vi "AddPropertyUnscale.vi"(0 "Data":T1={"Ref Cluster"={"String"=refnum, "U8"=refnum, "I8"=refnum, "U32"=refnum, "I32"=refnum, "U64"=refnum, "I64"=refnum, "Ring"=refnum, "DBL"=refnum, "Add"=refnum, "Remove"=refnum, "Property tree"=refnum}, "JSON Text"="", "Original JSON Text"="", "Caps"={"properties"=[], "physical channels"=[], "registers"=[], "scales"=[], "enums"=[], "productName"=""}, "SLSC Output Tree"=[], "Ref Index and Control Type"={"index"=0, "Datatype"=""}, "Selected Type and name"={"Selected Type"=enum."Property", "Selected Property Name"="Device/Properties/NI.Debug.ScratchU32.Min10Max20"}, "Update whole Tree?"=FALSE}, 1 "Scale method":string, 2 "Bitfield":string="DebugScratch8/ScratchI8", 5 "error in":errorcluster, 6 "Type&Value":cluster{"type":string, "Variant":variant}) -> (14 "Variant":variant, 19 "error out":errorcluster)   [LabVIEW 2017]
uses:
  <vilib>/Utility/Data Type/NI_Data Type.lvlib
  Ctrl/TableScale.ctl
  API/Scale/Scale.lvlib
  Ctrl/Coercion.ctl
  Ctrl/PolynomialScale.ctl
  Ctrl/LinearScale.ctl
  API/Bitfield/Bitfield.lvlib
  API/Scale/Unscale(Linear).vi
  API/Scale/Unscale(Table).vi
  API/Scale/Unscale(Polynomial).vi
  Ctrl/ScaleType.ctl
  Ctrl/Property.ctl
  Ctrl/PhysicalChannel.ctl
  Ctrl/Bitfield.ctl
  Ctrl/Register.ctl
  Ctrl/Scale.ctl
  Ctrl/EnumValue.ctl
  Ctrl/Enum.ctl
  Ctrl/Caps.ctl
  Ctrl/Data.ctl
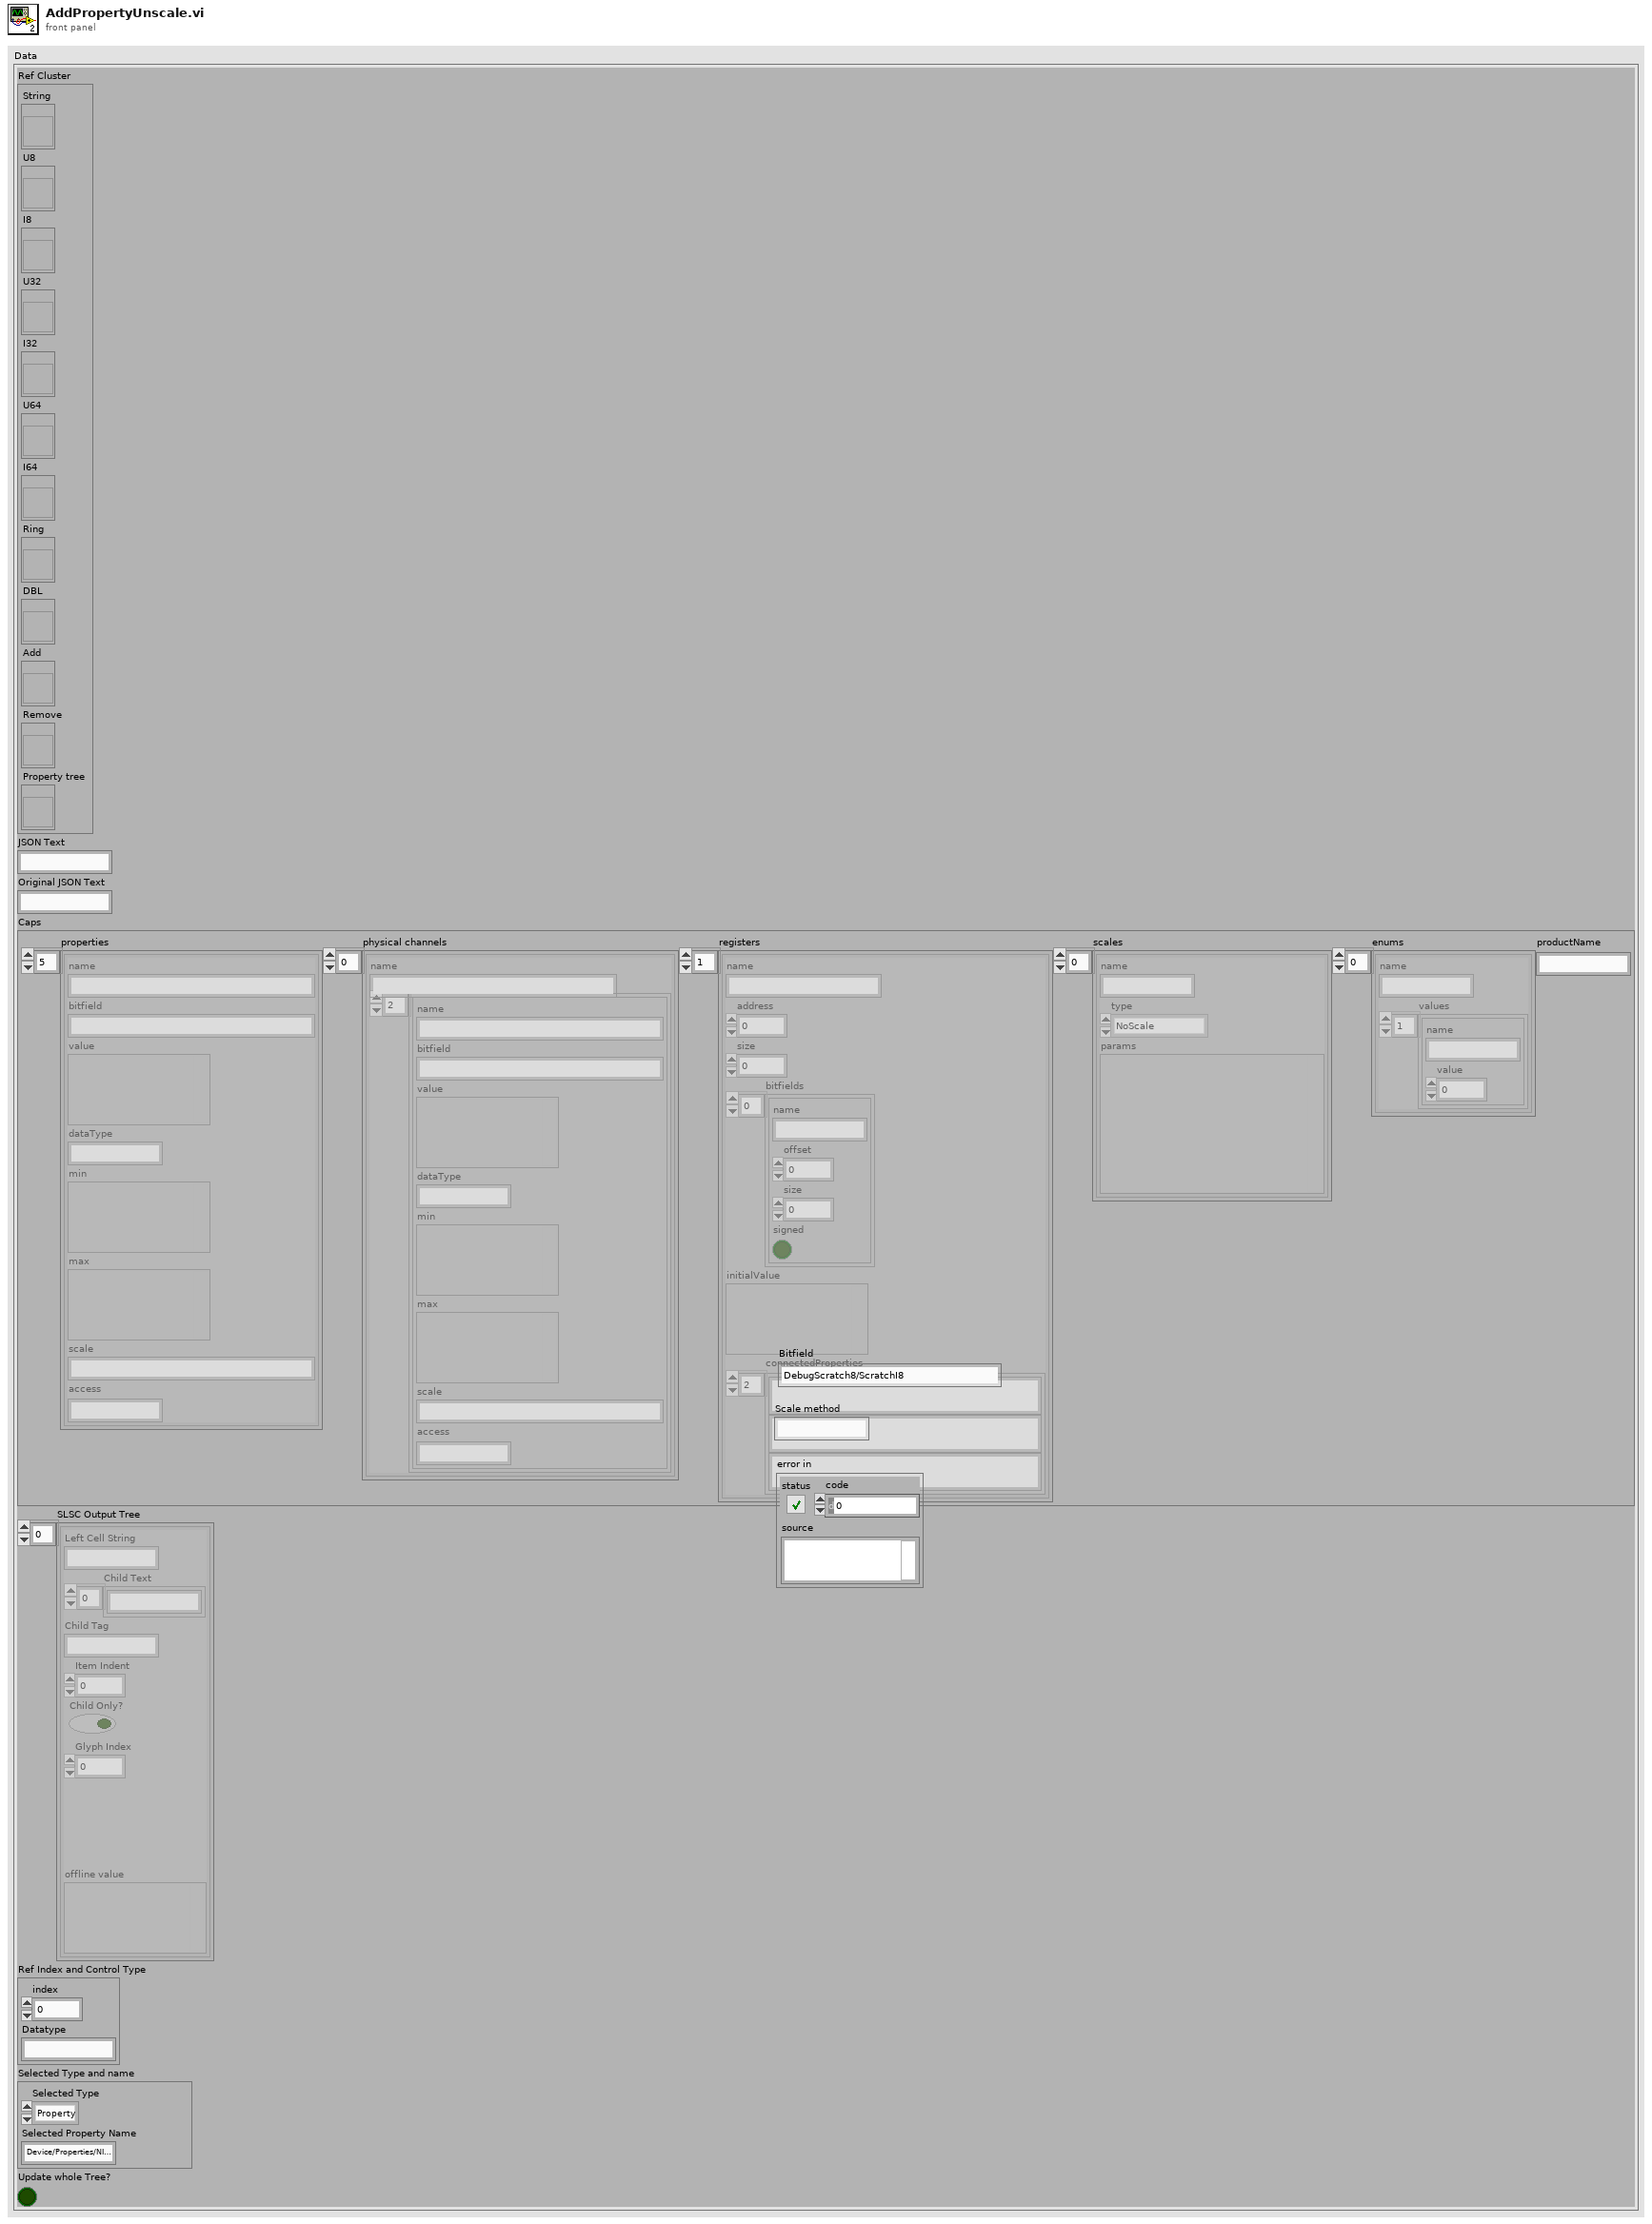
[diagram p1: front panel]
types:
  T1 = typedef "Data.ctl" = cluster{"Ref Cluster":cluster{"String":refnum<vi>, "U8":refnum<vi>, "I8":refnum<vi>, "U32":refnum<vi>, "I32":refnum<vi>, "U64":refnum<vi>, "I64":refnum<vi>, "Ring":refnum<vi>, "DBL":refnum<vi>, "Add":refnum<vi>, "Remove":refnum<vi>, "Property tree":refnum<vi>}, "JSON Text":string, "Original JSON Text":string, "Caps":T2, "SLSC Output Tree":cluster{"Left Cell String":string, "Child Text":string[], "Child Tag":string, "Item Indent":i32, "Child Only?":bool, "Glyph Index":i32, "offline value":variant}[], "Ref Index and Control Type":cluster{"index":i32, "Datatype":string}, "Selected Type and name":cluster{"Selected Type":enum16{"Property", "Physical Channel", "Other"}, "Selected Property Name":string}, "Update whole Tree?":bool}
  T2 = typedef "Caps.ctl" = cluster{"properties":T3[], "physical channels":T4[], "registers":T5[], "scales":T7[], "enums":T9[], "productName":string}
  T3 = typedef "Property.ctl" = cluster{"name":string, "bitfield":string, "value":variant, "dataType":string, "min":variant, "max":variant, "scale":string, "access":string}
  T4 = typedef "PhysicalChannel.ctl" = cluster{"name":string, "properties":T3[]}
  T5 = typedef "Register.ctl" = cluster{"name":string, "address":i32, "size":i32, "bitfields":T6[], "initialValue":variant, "connectedProperties":string[]}
  T6 = typedef "Bitfield.ctl" = cluster{"name":string, "offset":i32, "size":i32, "signed":bool}
  T7 = typedef "Scale.ctl" = cluster{"name":string, "type":T8, "params":variant}
  T8 = typedef "ScaleType.ctl" = enum16{"NoScale", "Table", "Polynomial", "Linear"}
  T9 = typedef "Enum.ctl" = cluster{"name":string, "values":T10[]}
  T10 = typedef "EnumValue.ctl" = cluster{"name":string, "value":i32}
  T11 = typedef "NI_Data Type.lvlib/Data Type.ctl" = enum8{"Invalid Type", "Void", "I8", "I16", "I32", "I64", "U8", "U16", "U32", "U64", "Single Float", "Double Float", "Extended Float", "Single Complex", "Double Complex", "Extended Complex", "Enum U8", "Enum U16", "Enum U32", "Enum U64", "Single Float With Unit", "Double Float With Unit", "Extended Float With Unit", "Single Complex with Unit", "Double Complex with Unit", "Extended Complex with Unit", "Boolean", "String", "Path", "Picture", "Tag", "Array", "Cluster", "Variant", "LV Variant", "Waveform", "Timestamp", "Digital Waveform", "Digital Data", "ExpressData", "Refnum", "External Data", "VI", "Poly VI", "LabVIEW Class Instance", "Fixed Point"}
  T12 = typedef "TableScale.ctl" = cluster{"name":string, "coercion":string, "table":cluster{"scaled":dbl, "unscaled":dbl}[]}
  T13 = typedef "Coercion.ctl" = enum16{"Strict", "RoundToNearest", "Interpolate"}
  T14 = typedef "PolynomialScale.ctl" = cluster{"name":string, "forwardCoeffs":dbl[], "reverseCoeffs":dbl[]}
  T15 = typedef "LinearScale.ctl" = cluster{"name":string, "m":dbl, "b":dbl}
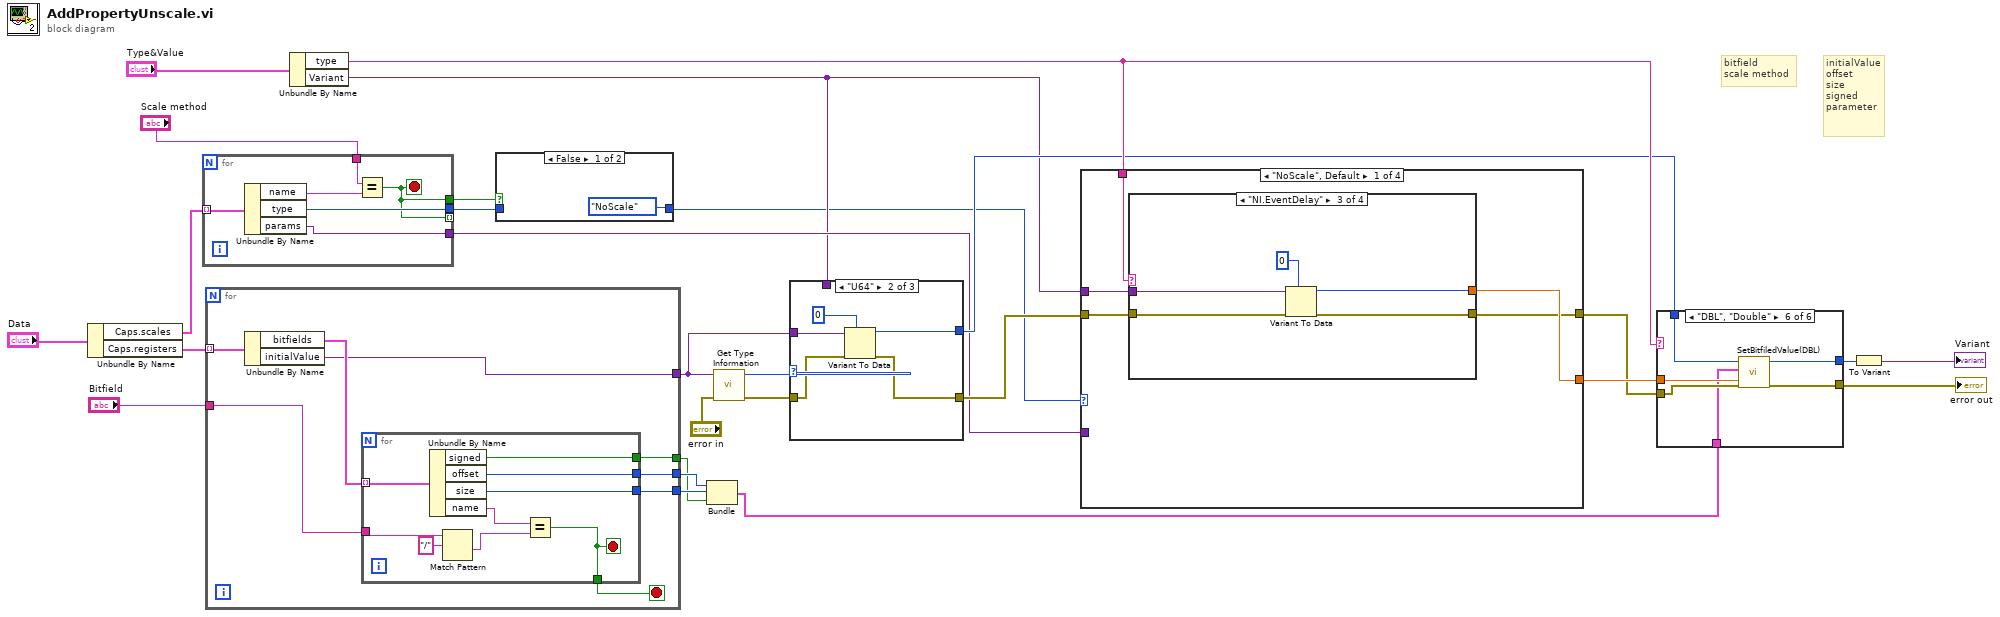
[diagram p0: block diagram]
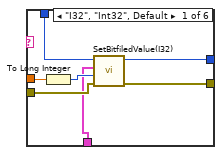
[diagram p3: hidden frame]
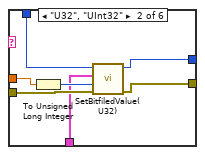
[diagram p4: hidden frame]
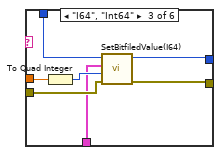
[diagram p5: hidden frame]
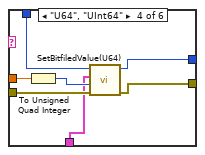
[diagram p6: hidden frame]
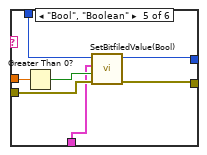
[diagram p7: hidden frame]
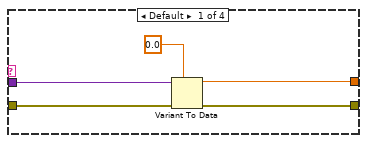
[diagram p8: hidden frame]
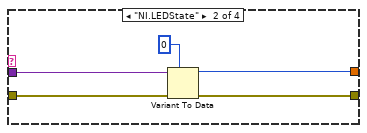
[diagram p9: hidden frame]
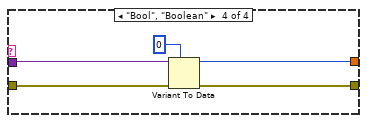
[diagram p10: hidden frame]
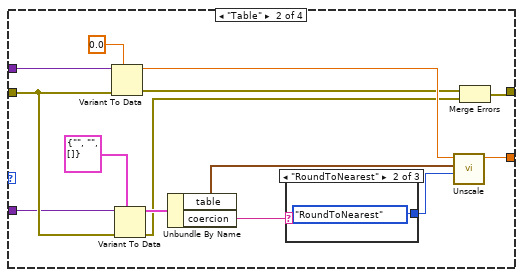
[diagram p11: hidden frame]
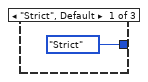
[diagram p12: hidden frame]
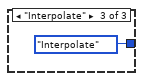
[diagram p13: hidden frame]
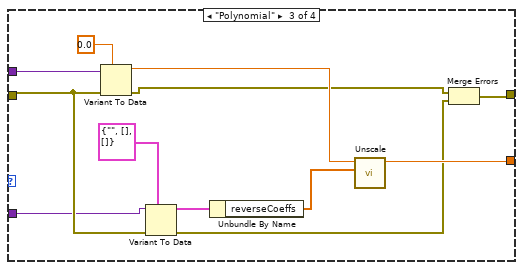
[diagram p14: hidden frame]
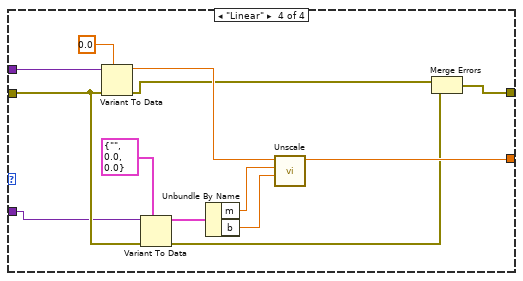
[diagram p15: hidden frame]
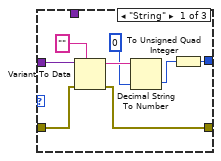
[diagram p16: hidden frame]
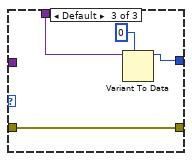
[diagram p17: hidden frame]
diagram:
  # "bitfield\nscale method"
  # "initialValue\noffset\nsize\nsigned\nparameter"
  n1 = Unbundle By Name("Data") -> ("Caps.scales"=w12:T7[], "Caps.registers"=w14:T5[])
  n2 = for {
    tunnel: w12 -> [w33] mode=indexing
    tunnel: "Scale method" -> [w31]
    tunnel: [w30] -> w2 if=w28
    tunnel: [w29] -> w10
    tunnel: [w28] -> _ mode=indexing
    tunnel: [w28] -> w3
    stop <- w28 stop-if-true
    n3 = Unbundle By Name(w33) -> ("name"=w32:string, "type"=w30:T8, "params"=w29:variant)
    n4 = Equal?(x=w31, y=w32) -> (x = y?=w28:bool)
  }
  n5 = for {
    tunnel: w14 -> [w41] mode=indexing
    tunnel: "Bitfield" -> [w39]
    tunnel: [w37] -> w7
    tunnel: [w36] -> w9
    tunnel: [w35] -> w8
    tunnel: [w34] -> w11
    stop <- w38 stop-if-true
    n6 = Unbundle By Name(w41) -> ("bitfields"=w40:T6[], "initialValue"=w34:variant)
    n7 = for {
      tunnel: w40 -> [w50] mode=indexing
      tunnel: w39 -> [w43]
      tunnel: [w48] -> w38
      tunnel: [w47] -> w37
      tunnel: [w46] -> w36
      tunnel: [w45] -> w35
      stop <- w48 stop-if-true
      n8 = Unbundle By Name(w50) -> ("signed"=w47:bool, "offset"=w46:i32, "size"=w45:i32, "name"=w49:string)
      n9 = Match Pattern(string=w43, regular expression="/") -> (after substring=w44:string)  [unwired: 1 in, 3 out]
      n10 = Equal?(x=w49, y=w44) -> (x = y?=w48:bool)
    }
  }
  n11 = Unbundle By Name("Type&Value") -> ("type"=w24:string, "Variant"=w4:variant)
  n12 = case shown="False" w3 {
    tunnel: w2 -> [_ w52]
    tunnel: [ScaleType."NoScale" ("type") w52] -> w1
    frame False {
    }
    frame True {
    }
  }
  n13 = Bundle("offset"=w9, "size"=w8, "signed"=w7) -> (w21:cluster{"offset":i32, "size":i32, "signed":bool})  [unwired: 1 in]
  n14 = call <vilib>:"Get Type Information.vi"("error in (no error)"="error in", "Variant"=w11) -> ("error out"=w22:errorcluster, "Type"=w23:T11)  [unwired: 5 in, 3 out]
  n15 = case shown="\"U64\"" w23 {
    tunnel: [w58 w64 w68] -> w20
    tunnel: w11 -> [w53 w61 _]
    tunnel: w22 -> [w55 w63 w69]
    tunnel: [w54 w62 w69] -> w17
    tunnel: w4 -> [_ _ w66]
    frame "String" {
      n16 = Variant To Data(error in=w55, type="", Variant=w53) -> (data=w59:string, error out=w54:errorcluster)
      n17 = Decimal String To Number(string=w59, default (0L)=u64 0 ("default (0 I32)")) -> (number=w57:u64)  [unwired: 1 in, 1 out]
      n18 = To Unsigned Quad Integer(1:w57) -> (0:w58:u64)
    }
    frame "U64" {
      n19 = Variant To Data(error in=w63, type=u64 0, Variant=w61) -> (data=w64:u64, error out=w62:errorcluster)
    }
    frame Default {
      n20 = Variant To Data(type=u64 0, Variant=w66) -> (data=w68:u64)  [unwired: 1 in, 1 out]
    }
  }
  n21 = case shown="\"NoScale\", Default" w1 {
    tunnel: w10 -> [_ w95 w112 w124]
    tunnel: w4 -> [w74 w103 w118 w135]
    tunnel: [w73 w100 w123 w129] -> w19
    tunnel: w17 -> [w72 w99 w116 w128]
    tunnel: [w71 w98 w115 w127] -> w16
    tunnel: w24 -> [w70 _ _ _]
    frame "NoScale", Default {
      n22 = case shown="\"NI.EventDelay\"" w70 {
        tunnel: w74 -> [w79 w83 w88 w90]
        tunnel: [w77 w81 w86 w92] -> w73
        tunnel: w72 -> [w76 w82 w87 w94]
        tunnel: [w75 w80 w85 w91] -> w71
        frame Default {
          n23 = Variant To Data(error in=w76, type=0.0, Variant=w79) -> (data=w77:dbl, error out=w75:errorcluster)
        }
        frame "NI.LEDState" {
          n24 = Variant To Data(error in=w82, type=0 ("Value"), Variant=w83) -> (data=w81:i32, error out=w80:errorcluster)
        }
        frame "NI.EventDelay" {
          n25 = Variant To Data(error in=w87, type=0 ("Value"), Variant=w88) -> (data=w86:i32, error out=w85:errorcluster)
        }
        frame "Bool", "Boolean" {
          n26 = Variant To Data(error in=w94, type=u16 0, Variant=w90) -> (data=w92:u16, error out=w91:errorcluster)
        }
      }
    }
    frame "Table" {
      n27 = Variant To Data(error in=w99, type=0.0, Variant=w103) -> (data=w101:dbl, error out=w97:errorcluster)
      n28 = Variant To Data(error in=w99, type=T12 {"name"="", "coercion"="", "table"=[]} ("TableScale"), Variant=w95) -> (data=w107:T12, error out=w96:errorcluster)
      n29 = Unbundle By Name(w107) -> ("table"=w105:cluster{"scaled":dbl, "unscaled":dbl}[], "coercion"=w106:string)
      n30 = case shown="\"RoundToNearest\"" w106 {
        tunnel: [Coercion."Strict" ("coercion") Coercion."RoundToNearest" ("coercion") Coercion."Interpolate" ("coercion")] -> w104
        frame "Strict", Default {
        }
        frame "RoundToNearest" {
        }
        frame "Interpolate" {
        }
      }
      n31 = call-poly "Unscale.vi"("coercion"=w104, "scales"=w105, "scale value"=w101) -> ("unscale value"=w100:dbl)  [unwired: 8 in]
      n32 = Merge Errors(w97, w96) -> (w98:errorcluster)
    }
    frame "Polynomial" {
      n33 = Variant To Data(error in=w116, type=0.0, Variant=w118) -> (data=w117:dbl, error out=w114:errorcluster)
      n34 = Variant To Data(error in=w116, type=T14 {"name"="", "forwardCoeffs"=[], "reverseCoeffs"=[]} ("PolynomialScale"), Variant=w112) -> (data=w121:T14, error out=w113:errorcluster)
      n35 = Unbundle By Name(w121) -> ("reverseCoeffs"=w120:dbl[])
      n36 = call-poly "Unscale.vi"("reverse coeffs"=w120, "scaled value"=w117) -> ("unscaled value"=w123:dbl)  [unwired: 9 in]
      n37 = Merge Errors(w114, w113) -> (w115:errorcluster)
    }
    frame "Linear" {
      n38 = Variant To Data(error in=w128, type=0.0, Variant=w135) -> (data=w134:dbl, error out=w126:errorcluster)
      n39 = Variant To Data(error in=w128, type=T15 {"name"="", "m"=0.0, "b"=0.0} ("LinearScale"), Variant=w124) -> (data=w132:T15, error out=w125:errorcluster)
      n40 = Unbundle By Name(w132) -> ("m"=w131:dbl, "b"=w130:dbl)
      n41 = call-poly "Unscale.vi"("offset"=w130, "multiplier"=w131, "scaled value"=w134) -> ("unscaled value"=w129:dbl)  [unwired: 8 in]
      n42 = Merge Errors(w126, w125) -> (w127:errorcluster)
    }
  }
  n43 = case shown="\"DBL\", \"Double\"" w24 {
    tunnel: w21 -> [w137 w144 w151 w158 w165 w172]
    tunnel: w20 -> [w143 w150 w157 w163 w171 w177]
    tunnel: w19 -> [w142 w149 w156 w164 w170 w176]
    tunnel: [w140 w147 w154 w161 w168 w175] -> w18
    tunnel: w16 -> [w139 w146 w153 w160 w167 w174]
    tunnel: [w138 w145 w152 w159 w166 w173] -> w27
    frame "I32", "Int32", Default {
      n44 = To Long Integer(number=w142) -> (32bit integer=w141:i32)
      n45 = call "SetBitfiledValue(I32).vi"("error in (no error)"=w139, "bitfield value"=w141, "bitfield caps"=w137, "original value"=w143) -> ("error out"=w138:errorcluster, "update value"=w140:u64)  [unwired: 6 in]
    }
    frame "U32", "UInt32" {
      n46 = To Unsigned Long Integer(number=w149) -> (unsigned 32bit integer=w148:u32)
      n47 = call "SetBitfiledValue(U32).vi"("error in (no error)"=w146, "bitfield value"=w148, "bitfield caps"=w144, "original value"=w150) -> ("error out"=w145:errorcluster, "update value"=w147:u64)  [unwired: 6 in]
    }
    frame "I64", "Int64" {
      n48 = To Quad Integer(1:w156) -> (0:w155:i64)
      n49 = call "SetBitfiledValue(I64).vi"("error in (no error)"=w153, "bitfield value"=w155, "bitfield caps"=w151, "original value"=w157) -> ("error out"=w152:errorcluster, "update value"=w154:u64)  [unwired: 6 in]
    }
    frame "U64", "UInt64" {
      n50 = To Unsigned Quad Integer(1:w164) -> (0:w162:u64)
      n51 = call "SetBitfiledValue(U64).vi"("error in (no error)"=w160, "bitfield value"=w162, "bitfield caps"=w158, "original value"=w163) -> ("error out"=w159:errorcluster, "update value"=w161:u64)  [unwired: 6 in]
    }
    frame "Bool", "Boolean" {
      n52 = Greater Than 0?(x=w170) -> (x > 0?=w169:bool)
      n53 = call "SetBitfiledValue(Bool).vi"("error in (no error)"=w167, "bitfield value"=w169, "bitfield caps"=w165, "original value"=w171) -> ("error out"=w166:errorcluster, "update value"=w168:u64)  [unwired: 6 in]
    }
    frame "DBL", "Double" {
      n54 = call "SetBitfiledValue(DBL).vi"("error in (no error)"=w174, "bitfield value"=w176, "bitfield caps"=w172, "original value"=w177) -> ("error out"=w173:errorcluster, "update value"=w175:u64)  [unwired: 6 in]
    }
  }
  "error out" <- w27
  n55 = To Variant(anything=w18) -> (Variant=→"Variant":variant)
